vi "SDSU_MemDump.vi"(7 "maxloc":i16, 8 "error in (no error)":errorcluster, 9 "args":string, 10 "board dest":i16, 11 "refnum":i32) -> (0 "error out":errorcluster, 2 "mem":string)   [LabVIEW 2016]
panel:
  in  "Array":string[](array[string])=["Y", "X"]
  out "fd out":i32
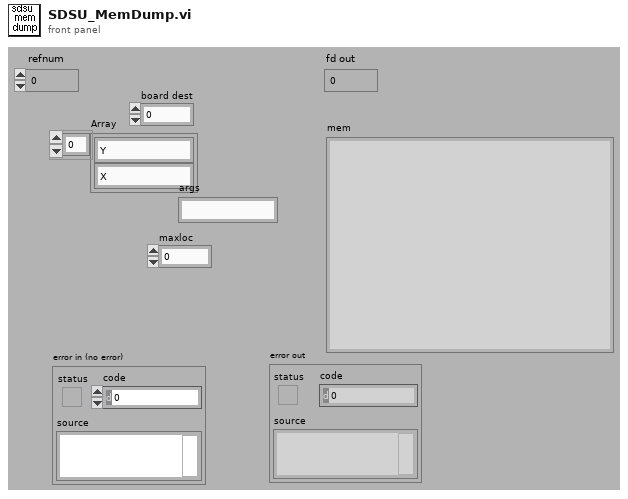
[diagram p1: front panel]
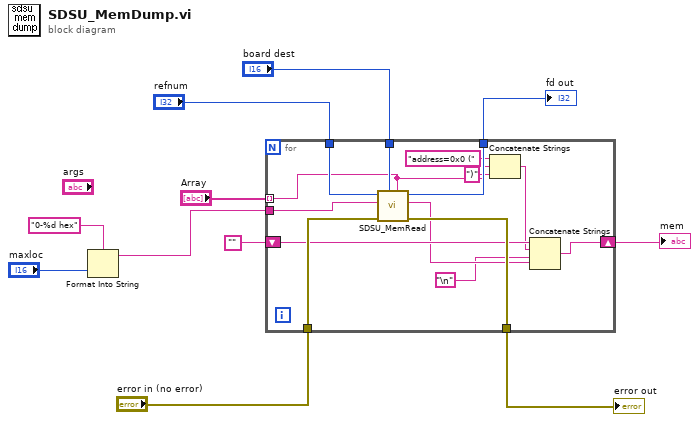
[diagram p0: block diagram]
diagram:
  n1 = Format Into String(format string="0-%d hex", "maxloc") -> (resulting string=w1:string)  [unwired: 2 in, 1 out]
  n2 = for {
    tunnel: "refnum" -> [w25]
    tunnel: [w24] -> w10
    tunnel: "error in (no error)" -> [w23]
    tunnel: [w22] -> w8
    shift-right: [w20] -> w4
    shift-left: "" -> [w19]
    tunnel: "Array" -> [w15] mode=indexing
    tunnel: "board dest" -> [w21]
    tunnel: w1 -> [w17]
    n3 = call "SDSU_MemRead.vi"("type"=w15, "board dest"=w21, "error in (no error)"=w23, "memin"=w17, "fd"=w25) -> ("error out"=w22:errorcluster, "values"=w18:string, "fd out"=w24:i32)  [unwired: 4 out]
    n4 = Concatenate Strings("address=0x0 (" ("string"), w15, ")" ("string")) -> (w13:string)
    n5 = Concatenate Strings(w19, w13, "\n", w18) -> (w20:string)
  }
  "mem" <- w4
  "error out" <- w8
  "fd out" <- w10
